vi "recipeScript checkTableParam.vi"(8 "error in (no error)":errorcluster, 10 "newVal":string[][](array[string]), 11 "tableRefNum":refnum<vi>) -> (0 "error out":errorcluster, 3 "valid":bool)   [LabVIEW 2018]
uses:
  <vilib>/Utility/miscctls.llb/LVRowAndColumnTypeDef.ctl
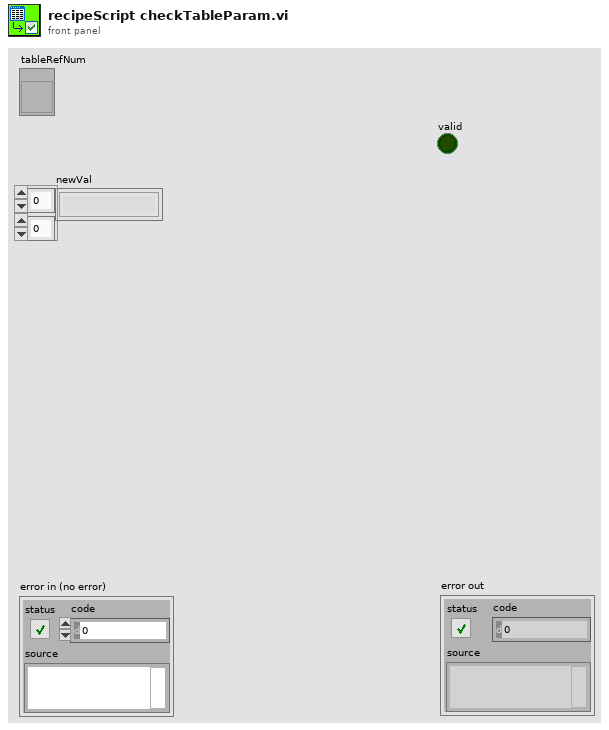
[diagram p1: front panel]
types:
  T1 = typedef "LVRowAndColumnTypeDef.ctl" = cluster{"Row":i32, "Column":i32}
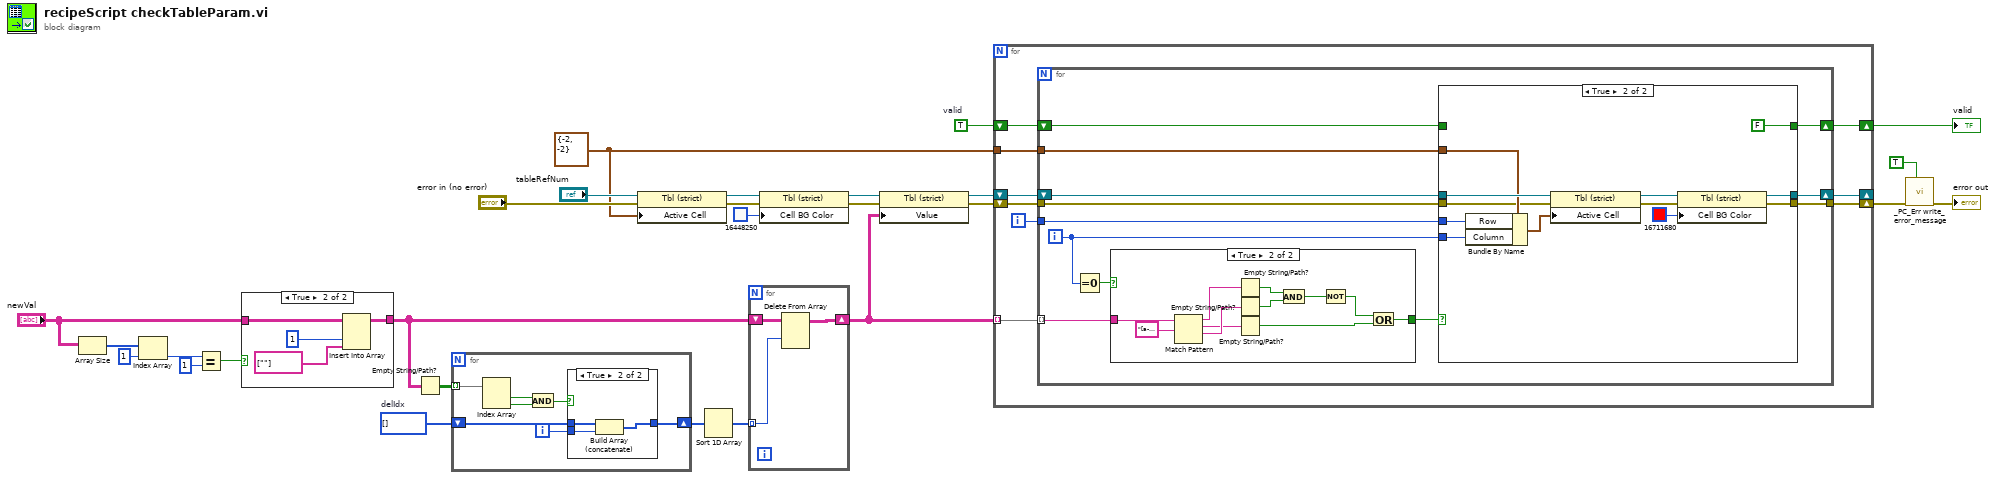
[diagram p0: block diagram]
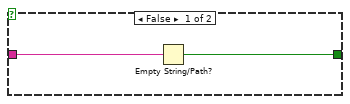
[diagram p2: hidden frame]
diagram:
  w8 = TRUE  # valid
  w2 = T1 {"Row"=-2, "Column"=-2} ("Active Cell:Active Cell")
  w20 = i32[] []  # delIdx
  n1 = Array Size(array="newVal") -> (size(s)=w27:i32[])
  n2 = Index Array(array=w27, index=1) -> (element=w25:i32)
  n3 = Equal?(x=w25, y=1) -> (x = y?=w22:bool)
  n4 = case shown="True" w22 {
    tunnel: "newVal" -> [w28 w32]
    tunnel: [w28 w29] -> w18
    frame False {
    }
    frame True {
      n5 = Insert Into Array(array=w32, index (col)=1 ("disabled index (row)"), new element=string[] [""] ("new element/subarray")) -> (w29:string[][])  [unwired: 1 in]
    }
  }
  n6 = Empty String/Path?(string/path=w18) -> (empty?=w21:bool[][])
  n7 = for {
    tunnel: w21 -> [w39] mode=indexing
    shift-right: [w33] -> w19
    shift-left: w20 -> [w35]
    i -> [w34]
    n8 = Index Array(array=w39) -> (element #1=w38:bool, element #2=w37:bool)  [unwired: 2 in]
    n9 = And(x=w38, y=w37) -> (x .and. y?=w36:bool)
    n10 = case shown="True" w36 {
      tunnel: w35 -> [w40 w43]
      tunnel: w34 -> [_ w42]
      tunnel: [w40 w41] -> w33
      frame False {
      }
      frame True {
        n11 = Build Array (concatenate)(w43, w42) -> (w41:i32[])
      }
    }
  }
  n12 = property class="Tbl (strict)"(reference="tableRefNum", error in="error in (no error)", "Active Cell"=w2) -> (reference out=w12:refnum<vi>, error out=w14:errorcluster)
  n13 = Sort 1D Array(array=w19) -> (sorted array=w17:i32[])
  n14 = for {
    shift-right: [w44] -> w5
    shift-left: w18 -> [w45]
    tunnel: w17 -> [w46] mode=indexing
    n15 = Delete From Array(array=w45, index (row)=w46) -> (array with subset deleted=w44:string[][])  [unwired: 2 in, 1 out]
  }
  n16 = property class="Tbl (strict)"(reference=w12, error in=w14, "Cell BG Color"=u32 16448250) -> (reference out=w11:refnum<vi>, error out=w10:errorcluster)
  n17 = property class="Tbl (strict)"(reference=w11, error in=w10, "Value"=w5) -> (reference out=w4:refnum<vi>, error out=w3:errorcluster)
  n18 = for {
    tunnel: w5 -> [w55] mode=indexing
    tunnel: w2 -> [w53]
    shift-right: [w51] -> w1
    shift-left: w3 -> [w52]
    shift-right: [w49] -> w9
    shift-left: w8 -> [w50]
    shift-right: [w48] -> _
    shift-left: w4 -> [w47]
    i -> [w54]
    n19 = for {
      tunnel: w55 -> [w61] mode=indexing
      tunnel: w54 -> [w67]
      tunnel: w53 -> [w65]
      tunnel: w52 -> [w64]
      tunnel: [w63] -> w51
      shift-right: [w58] -> w49
      shift-left: w50 -> [w59]
      shift-right: [w56] -> w48
      shift-left: w47 -> [w66]
      i -> [w57]
      n20 = Equal To 0?(x=w57) -> (x = 0?=w62:bool)
      n21 = case shown="True" w62 {
        tunnel: w61 -> [w69 w80]
        tunnel: [w68 w70] -> w60
        frame False {
          n22 = Empty String/Path?(string/path=w69) -> (empty?=w68:bool)
        }
        frame True {
          n23 = Match Pattern(string=w80, regular expression="[a-zA-Z][a-zA-Z\\_0-9]*") -> (before substring=w78:string, match substring=w74:string, after substring=w77:string)  [unwired: 1 in, 1 out]
          n24 = Empty String/Path?(string/path=w78) -> (empty?=w76:bool)
          n25 = Empty String/Path?(string/path=w77) -> (empty?=w75:bool)
          n26 = Empty String/Path?(string/path=w74) -> (empty?=w71:bool)
          n27 = And(x=w76, y=w75) -> (x .and. y?=w73:bool)
          n28 = Not(x=w73) -> (.not. x?=w72:bool)
          n29 = Or(x=w72, y=w71) -> (x .or. y?=w70:bool)
        }
      }
      n30 = case shown="True" w60 {
        tunnel: w67 -> [_ w85]
        tunnel: w57 -> [_ w84]
        tunnel: w66 -> [w82 w95]
        tunnel: w65 -> [_ w94]
        tunnel: w64 -> [w83 w89]
        tunnel: [w83 w88] -> w63
        tunnel: [w81 FALSE] -> w58
        tunnel: w59 -> [w81 _]
        tunnel: [w82 w86] -> w56
        frame False {
        }
        frame True {
          n31 = Bundle By Name(cluster=w94, "Row"=w85, "Column"=w84) -> (w93:T1)
          n32 = property class="Tbl (strict)"(reference=w95, error in=w89, "Active Cell"=w93) -> (reference out=w91:refnum<vi>, error out=w90:errorcluster)
          n33 = property class="Tbl (strict)"(reference=w91, error in=w90, "Cell BG Color"=u32 16711680) -> (reference out=w86:refnum<vi>, error out=w88:errorcluster)
        }
      }
    }
  }
  "valid" <- w9
  n34 = call "_PC_Err write_error_message.vi"("show msg( T )"=TRUE ("skipWrong( T )"), "error in"=w1) -> ("error out"=→"error out":errorcluster)  [unwired: 9 in]
